vi "Build Object Dictionary.vi"(8 "error in (no error)":errorcluster, 11 "EDS in":refnum<class "EDS.lvclass">) -> (0 "error out":errorcluster, 3 "EDS out":refnum<class "EDS.lvclass">)   [LabVIEW 2024, in "EDS.lvlib" / "EDS.lvclass"]
uses:
  EDS.lvclass
  EDS.lvclass/EDS.ctl
  OD Section/Section.lvclass
  <vilib>/Utility/config.llb/NI_LVConfig.lvlib
  Object Dictionary/Object Dictionary.lvclass
  <vilib>/Utility/config.llb/Read Key (String).vi
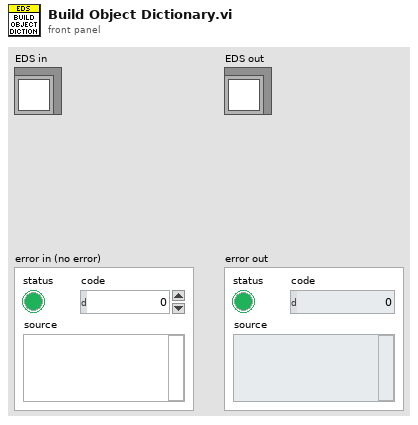
[diagram p1: front panel]
types:
  T1 = typedef "NI_LVConfig.lvlib/Config Data RefNum.ctl" = refnum<k1>
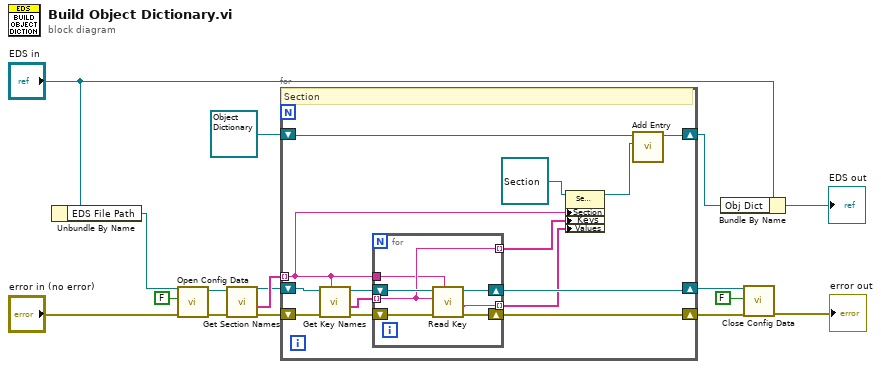
[diagram p0: block diagram]
diagram:
  n1 = Unbundle By Name("EDS in") -> ("EDS File Path"=w11:path)
  n2 = call <vilib>:"Open Config Data.vi"("error in (no error)"="error in (no error)", "create file if necessary (T)"=FALSE, "configuration file path"=w11) -> ("error out"=w1:errorcluster, "refnum"=w2:T1)  [unwired: 6 in, 1 out]
  n3 = call <vilib>:"Get Section Names.vi"("error in (no error)"=w1, "refnum"=w2) -> ("error out"=w4:errorcluster, "section names"=w13:string[], "refnum out"=w5:T1)  [unwired: 7 in]
  n4 = for {
    tunnel: w13 -> [w17] mode=indexing
    shift-right: [w27] -> w6
    shift-left: w4 -> [w30]
    shift-right: [w25] -> w7
    shift-left: w5 -> [w29]
    shift-right: [w22] -> w14
    shift-left: refnum<class "Object Dictionary.lvclass"> refnum ("Object Dictionary") -> [w21]
    # "Section"
    n5 = call <vilib>:"Get Key Names.vi"("section"=w17, "error in (no error)"=w30, "refnum"=w29) -> ("error out"=w28:errorcluster, "key names"=w24:string[], "refnum out"=w26:T1)  [unwired: 5 in, 1 out]
    n6 = for {
      shift-right: [w33] -> w27
      shift-left: w28 -> [w37]
      tunnel: w24 -> [w32] mode=indexing
      shift-right: [w35] -> w25
      shift-left: w26 -> [w36]
      tunnel: [w34] -> w19 mode=indexing
      tunnel: [w32] -> w18 mode=indexing
      tunnel: w17 -> [w31]
      n7 = call-poly <vilib>:"Read Key.vi"("section"=w31, "error in (no error)"=w37, "key"=w32, "refnum"=w36) -> ("error out"=w33:errorcluster, "value"=w34:string, "refnum out"=w35:T1)  [unwired: 4 in, 1 out]
    }
    n8 = property class="Section.lvclass"(reference=refnum<class "Section.lvclass"> refnum ("Object Entry"), "Section"=w17, "Keys"=w18, "Values"=w19) -> (reference out=w20:refnum<class "Section.lvclass">)  [unwired: 1 in, 1 out]
    n9 = call "Add Entry.vi"("Object Entry"=w20, "Object Dictionary in"=w21) -> ("Object Dictionary out"=w22:refnum<class "Object Dictionary.lvclass">)  [unwired: 9 in]
  }
  n10 = Bundle By Name(cluster="EDS in", "Obj Dict"=w14) -> (→"EDS out":refnum<class "EDS.lvclass">)
  n11 = call <vilib>:"Close Config Data.vi"("error in (no error)"=w6, "write file if changed (T)"=FALSE, "refnum"=w7) -> ("error out"=→"error out":errorcluster)  [unwired: 7 in, 1 out]
